vi "Finalize To Settings.vi"(8 "error in (no error)":errorcluster, 11 "Core Channels Configuration in":refnum<class "Channel Configuration.lvclass">) -> (0 "error out":errorcluster, 2 "settings":cluster{"key":string, "value":string}[](array[cluster]), 3 "Core Channels Configuration out":refnum<class "Channel Configuration.lvclass">)   [LabVIEW 2019, in "DSF Core.lvlib" / "Channel Configuration.lvclass"]
uses:
  Channel Configuration.lvclass
  Channel Configuration.lvclass/Channel Configuration.ctl
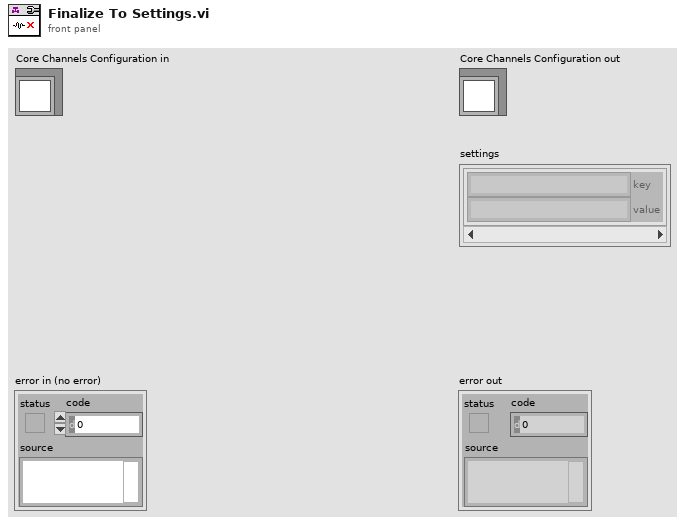
[diagram p1: front panel]
types:
  T1 = typedef "DSF Core.lvlib/DSF Version Info.ctl" = cluster{"major":u32, "minor":u32, "fix":u32, "build":string}
  T2 = typedef "DSF Core.lvlib/Channel Configuration.lvclass/Core Channel Configuration.ctl" = cluster{"name":string, "units":string, "engine data type":T3, "string data type":T3, "string offset":u64}
  T3 = typedef "DSF Core.lvlib/DSF Data Type.ctl" = enum8{"Bool", "SGL", "DBL", "I8", "I16", "I32", "I64", "U8", "U16", "U32", "U64"}
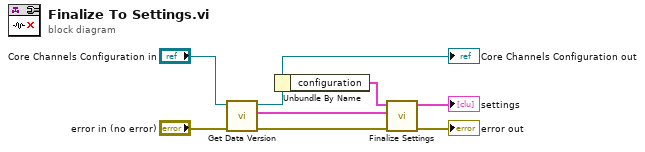
[diagram p0: block diagram]
diagram:
  n1 = call-dynamic "Get Data Version.vi"("error in (no error)"="error in (no error)", "Core Channels Configuration in"="Core Channels Configuration in") -> ("error out"=w6:errorcluster, "data version"=w4:T1, "Core Channels Configuration out"=w1:refnum<class "Channel Configuration.lvclass">)  [unwired: 7 in]
  "Core Channels Configuration out" <- w1
  n2 = Unbundle By Name(w1) -> ("configuration"=w3:T2)
  n3 = call "Finalize Settings.vi"("error in (no error)"=w6, "settings version"=w4, "configuration"=w3) -> ("error out"=→"error out":errorcluster, "settings"=→"settings":cluster{"key":string, "value":string}[])  [unwired: 6 in, 1 out]
